vi "host_chunk (2 DMA(.vi"() -> ()   [LabVIEW 2020]
doc: "This example demonstrates how to continuously acquire buffered voltage measurements using a DAQmx device.\n\nFor instructions on how to connect your signals to the DAQ device, refer to your device documentation."
uses:
  <vilib>/DAQmx/read.llb/DAQmx Read (Analog Wfm 1Chan NSamp).vi
  <vilib>/DAQmx/create/channels.llb/DAQmx Create Channel (AI-Voltage-Basic).vi
  <vilib>/DAQmx/configure/timing.llb/DAQmx Timing (Sample Clock).vi
  <vilib>/FPGAPlugInAG/cRIO-9040/niLvFpga_Open_cRIO-9040.vi
  <vilib>/rvi/interface/common/dynamic/niFpgaDynamicAddResources.vi
  <vilib>/Utility/error.llb/Error Cluster From Error Code.vi
  <vilib>/rvi/errors/niLvFpgaAdjustHostInterfaceError.vi
  <vilib>/FPGAPlugInAG/Dynamic/niLvFpga_Run_Dynamic.vi
  <vilib>/RVI Host/nirviSupport.llb/nirviErrorClusterFromErrorCode.vi
  <vilib>/DAQmx/miscellaneous.llb/DAQmx Fill In Error Info.vi
  <vilib>/FPGAPlugInAG/Dynamic/niLvFpga_Close_Dynamic.vi
  <vilib>/rvi/interface/nirviOpenFPGA/nirviOpenFPGA.xnode
  FPGA Bitfiles/testDMA_9040_chunk_v1002.lvbitx
  <vilib>/rvi/interface/nirviReadWriteControl/nirviReadWriteControl.xnode
  <vilib>/rvi/interface/nirviMethod/nirviMethod.xnode
  <vilib>/rvi/interface/nirviCloseFPGA/nirviCloseFPGA.xnode
  <resource>/objmgr/daqmx.rc
  <vilib>/rvi/interface/Simulation/niFpgaSimulationCallBeginRW.vi
  <vilib>/rvi/errors/niLvFpgaMergeErrorWithErrorCode.vi
  NiFpgaLv.dll
  <vilib>/FPGAPlugInAG/Dynamic/niLvFpga_WriteFifo_Dynamic.vi
  <vilib>/FPGAPlugInAG/Dynamic/niLvFpga_ReadFifo_Dynamic.vi
  <vilib>/rvi/interface/nirviMethod/StockFPGA_InlinedMethodWaitForSingleIRQ.vi
  <vilib>/FPGAPlugInAG/Dynamic/niLvFpga_WaitOnIrq_Dynamic.vi
  <vilib>/FPGAPlugInAG/Dynamic/niLvFpga_AcknowledgeIrq_Dynamic.vi
panel:
  out "dma read time uS 2":u32
  out "write DMA timeout count 2":i16
  out "dma read time uS":u32
  out "AvailSampPerChan":u32
  out "write DMA timeout count":i16
  out "uS elapsed":cluster{u32, u32}(graph)
  out "Timed Out":bool
  out "error out":errorcluster
  in  "Stop":bool
  out "Waveform Graph":dbl[][](graph)
  in  "Number of Samples":i32=100
  in  "Sample Rate":dbl=1000.0
  in  "Sample Clock Source":tag="OnboardClock"
  in  "Terminal Configuration":i32(ring)=-1 items=["default"=-1, "RSE"=10083, "NRSE"=10078, "Differential"=10106, "Pseudodifferential"=12529]
  in  "Max Voltage":dbl=5.0
  in  "Min Voltage":dbl=-5.0
  in  "Physical Channel":tag="Mod1/ai0"
  out "Actual Sample Rate":dbl=1000.0 format="%0.2f"
  # "Channel Settings"
  # "Acquired Data"
  # "Timing Settings"
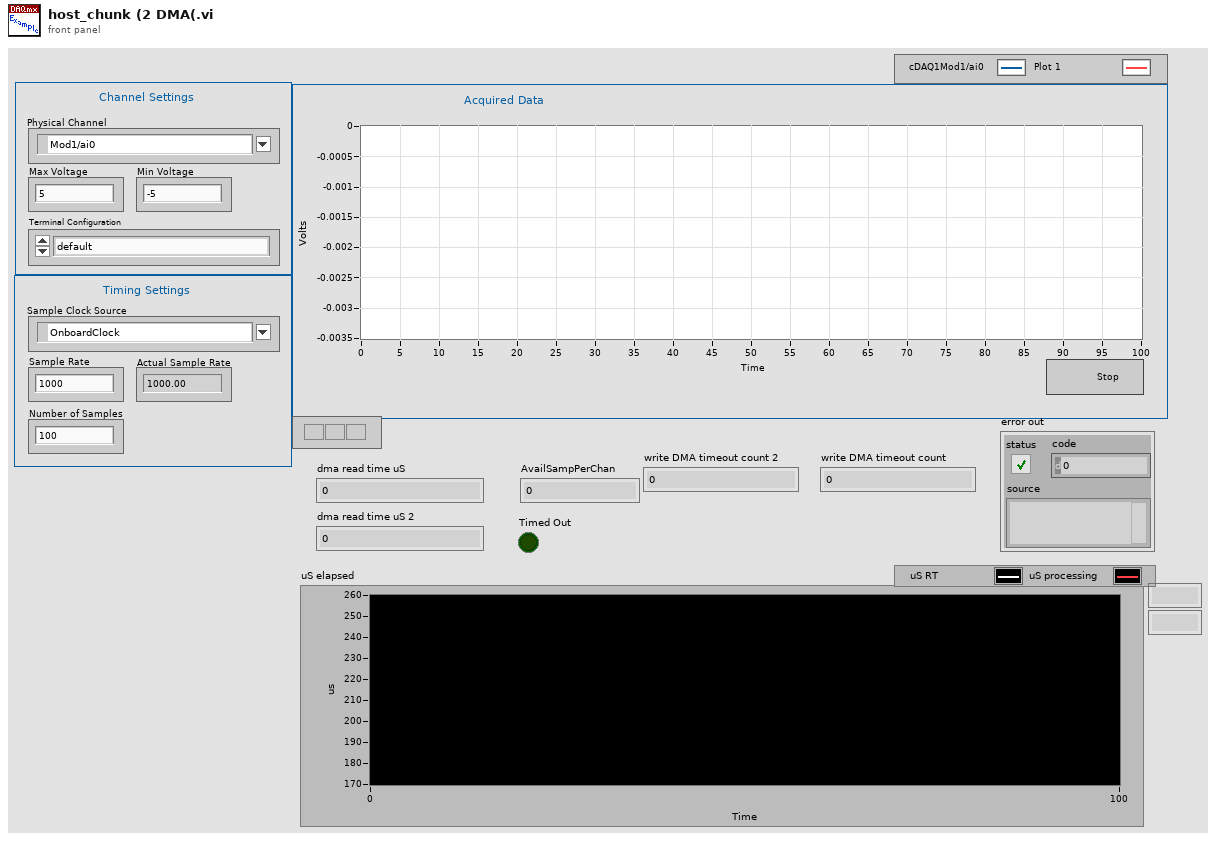
[diagram p1: front panel]
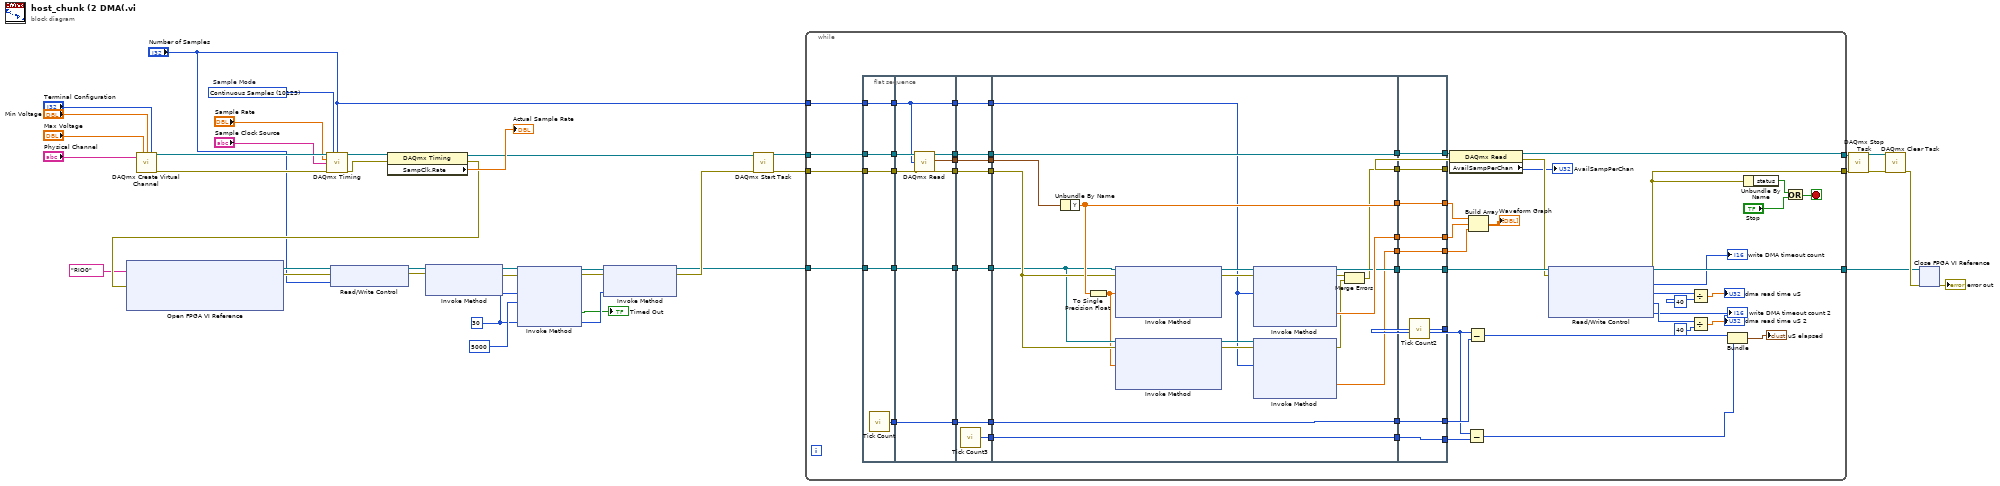
[diagram p0: block diagram]
diagram:
  w5 = u8 30 ("IRQ Number (0)")
  w36 = 10123 items=["Finite Samples"=10178, "Continuous Samples"=10123, "Hardware Timed Single Point"=12522]  # Sample Mode
  n1 = call-poly <vilib>:"DAQmx Create Virtual Channel.vi"("maximum value"="Max Voltage", "minimum value"="Min Voltage", "input terminal configuration"="Terminal Configuration", "physical channels"="Physical Channel") -> ("task out"=w34:refnum<k21>, "error out"=w35:errorcluster)  [unwired: 10 in]
  n2 = call-poly <vilib>:"DAQmx Timing.vi"("task/channels in"=w34, "sample mode"=w36, "samples per channel"="Number of Samples", "rate"="Sample Rate", "source"="Sample Clock Source", "error in"=w35) -> ("task out"=w38:refnum<k21>, "error out"=w37:errorcluster)  [unwired: 8 in]
  n3 = property class="DAQmx Timing"(reference=w38, error in=w37) -> (reference out=w17:refnum<k21>, error out=w18:errorcluster, "SampClk.Rate"=→"Actual Sample Rate":dbl)
  n4 = xnode "Open FPGA VI Reference"("error in"=w18, "resource name"=tag "RIO0") -> ("FPGA VI Reference Out"=w15:refnum<k20>, "error out"=w16:errorcluster)
  n5 = xnode "Read/Write Control"("FPGA VI Reference In"=w15, "error in"=w16, "number of samples"="Number of Samples") -> ("FPGA VI Reference Out"=w12:refnum<k20>, "error out"=w11:errorcluster)
  n6 = xnode "Invoke Method"("FPGA VI Reference In"=w12, "error in"=w11) -> ("FPGA VI Reference Out"=w10:refnum<k20>, "error out"=w9:errorcluster)  [unwired: 1 in]
  n7 = xnode "Invoke Method"("FPGA VI Reference In"=w10, "error in"=w9, "IRQ Number(s)"=w5, "Timeout (ms)"=5000) -> ("FPGA VI Reference Out"=w8:refnum<k20>, "error out"=w7:errorcluster, "Timed Out"=→"Timed Out":bool)  [unwired: 1 out]
  n8 = xnode "Invoke Method"("FPGA VI Reference In"=w8, "error in"=w7, "IRQ Number(s)"=w5) -> ("FPGA VI Reference Out"=w2:refnum<k20>, "error out"=w3:errorcluster)
  n9 = call <vilib>:"DAQmx Start Task.vi"("task/channels in"=w17, "error in"=w3) -> ("task out"=w33:refnum<k21>, "error out"=w32:errorcluster)  [unwired: 12 in]
  n10 = while {
    tunnel: w33 -> [w97]
    tunnel: w32 -> [w92]
    tunnel: [w74] -> w24
    tunnel: [w77] -> w23
    tunnel: "Number of Samples" -> [w62]
    tunnel: w2 -> [w91]
    tunnel: [w78] -> w1
    stop <- w93 stop-if-true
    n11 = flat-sequence {
      tunnel: w97 -> [w102]
      tunnel: [w102] -> w67
      tunnel: [w101] -> w66
      tunnel: w92 -> [w101]
      tunnel: [w100] -> w65
      tunnel: w91 -> [w100]
      tunnel: [w99] -> w64
      tunnel: [w98] -> w63
      tunnel: w62 -> [w98]
      tunnel: w67 -> [w108]
      tunnel: [w108] -> w61
      tunnel: w66 -> [w107]
      tunnel: [w107] -> w59
      tunnel: w65 -> [w106]
      tunnel: [w106] -> w57
      tunnel: w64 -> [w105]
      tunnel: [w105] -> w55
      tunnel: [w104] -> w53
      tunnel: w63 -> [w103]
      tunnel: [w103] -> w51
      tunnel: w61 -> [w115]
      tunnel: [w115] -> w60
      tunnel: w59 -> [w114]
      tunnel: [w114] -> w58
      tunnel: w57 -> [w113]
      tunnel: [w113] -> w56
      tunnel: w55 -> [w112]
      tunnel: [w112] -> w54
      tunnel: w53 -> [w111]
      tunnel: [w111] -> w52
      tunnel: w51 -> [w110]
      tunnel: [w110] -> w50
      tunnel: [w109] -> w46
      tunnel: w60 -> [w126]
      tunnel: w58 -> [w122]
      tunnel: w56 -> [w121]
      tunnel: [w126] -> w86
      tunnel: [w119] -> w85
      tunnel: [w132] -> w84
      tunnel: [w131] -> w83
      tunnel: [w129] -> w82
      tunnel: [w128] -> w80
      tunnel: w54 -> [w128]
      tunnel: w52 -> [w127]
      tunnel: w50 -> [w117]
      tunnel: [w125] -> w47
      tunnel: w46 -> [w125]
      tunnel: [w120] -> w43
      tunnel: [w139] -> w87
      tunnel: [w140] -> w90
      tunnel: [w141] -> w89
      tunnel: [w142] -> w73
      tunnel: [w143] -> w96
      tunnel: w86 -> [w143]
      tunnel: w85 -> [w142]
      tunnel: w84 -> [w141]
      tunnel: w83 -> [w140]
      tunnel: w82 -> [w139]
      tunnel: [w138] -> w49
      tunnel: [w137] -> w81
      tunnel: w80 -> [w137]
      tunnel: [w136] -> w48
      tunnel: w47 -> [w136]
      tunnel: [w135] -> w44
      tunnel: w43 -> [w135]
      frame #0 {
        n12 = call "Tick Count"() -> ("Tick Count(uSec)"=w99:u32)
      }
      frame #1 {
        n13 = call-poly <vilib>:"DAQmx Read.vi"("task/channels in"=w108, "number of samples per channel"=w103, "error in"=w107) -> ("data"=w104:waveform(dbl))  [unwired: 10 in, 2 out]
      }
      frame #2 {
        n14 = call "Tick Count3"() -> ("Tick Count(uSec)"=w109:u32)
      }
      frame #3 {
        n15 = Unbundle By Name(w127) -> ("Y"=w131:dbl[])
        n16 = To Single Precision Float(number=w131) -> (single precision float=w116:sgl[])
        n17 = xnode "Invoke Method"("FPGA VI Reference In"=w121, "error in"=w122, "Data"=w116) -> ("FPGA VI Reference Out"=w134:refnum<k20>, "error out"=w133:errorcluster)  [unwired: 1 in, 1 out]
        n18 = xnode "Invoke Method"("FPGA VI Reference In"=w121, "error in"=w122, "Data"=w116) -> ("FPGA VI Reference Out"=w123:refnum<k20>, "error out"=w124:errorcluster)  [unwired: 1 in, 1 out]
        n19 = xnode "Invoke Method"("FPGA VI Reference In"=w134, "error in"=w133, "Number of Elements"=w117) -> ("FPGA VI Reference Out"=w129:refnum<k20>, "error out"=w130:errorcluster, "Data"=w132:sgl[])  [unwired: 1 in, 1 out]
        n20 = xnode "Invoke Method"("FPGA VI Reference In"=w123, "error in"=w124, "Number of Elements"=w117) -> ("error out"=w118:errorcluster, "Data"=w120:sgl[])  [unwired: 1 in, 2 out]
        n21 = Merge Errors(w130, w118) -> (w119:errorcluster)
      }
      frame #4 {
        n22 = call "Tick Count2"() -> ("Tick Count(uSec)"=w138:u32)
      }
    }
    n23 = property class="DAQmx Read"(reference=w96, error in=w73) -> (reference out=w74:refnum<k21>, error out=w72:errorcluster, "AvailSampPerChan"=→"AvailSampPerChan":u32)
    n24 = Subtract(x=w49, y=w48) -> (x-y=w45:u32)
    n25 = Subtract(x=w49, y=w81) -> (x-y=w79:u32)
    n26 = Build Array(w90, w89, w44) -> (→"Waveform Graph":dbl[][])
    n27 = xnode "Read/Write Control"("FPGA VI Reference In"=w87, "error in"=w72) -> ("FPGA VI Reference Out"=w78:refnum<k20>, "error out"=w77:errorcluster, "write DMA timeout count"=→"write DMA timeout count":i16, "dma read time ticks"=w70:u32, "dma read time ticks 2"=w41:u32, "write DMA timeout count 2"=→"write DMA timeout count 2":i16)
    n28 = Divide(x=w70, y=u32 40) -> (x/y=→"dma read time uS":dbl)
    n29 = Divide(x=w41, y=u32 40) -> (x/y=→"dma read time uS 2":dbl)
    n30 = Bundle(w79, w45) -> (→"uS elapsed":cluster{u32, u32})  [unwired: 1 in]
    n31 = Unbundle By Name(w77) -> ("status"=w94:bool)
    n32 = Or(x=w94, y="Stop") -> (x .or. y?=w93:bool)
  }
  n33 = call <vilib>:"DAQmx Stop Task.vi"("task/channels in"=w24, "error in"=w23) -> ("task out"=w21:refnum<k21>, "error out"=w22:errorcluster)  [unwired: 12 in]
  n34 = call <vilib>:"DAQmx Clear Task.vi"("task in"=w21, "error in"=w22) -> ("error out"=w20:errorcluster)  [unwired: 13 in]
  n35 = xnode "Close FPGA VI Reference"("FPGA VI Reference In"=w1, "error in"=w20) -> ("error out"=→"error out":errorcluster)
